vi "initialize.vi"(0 "HGF_Queue":refnum<class "HGF_Queue.lvclass">, 3 "initializationData":variant, 5 "error in (no error)":errorcluster, 7 "binaryString":string, 8 "I8 Array":i8[](array[numeric]), 9 "prependSize? (T)":bool, 11 "byteOrder (0:big-endian, network order)":T1(ring)) -> (14 "dup HGF_Queue":refnum<class "HGF_Queue.lvclass">, 17 "found?":bool, 19 "error out":errorcluster)   [LabVIEW 2014, in "HGF_BaseClasses.lvlib" / "HGF_Queue.lvclass"]
doc: "This is a dynamic dispatch VI to be implemented by child classes to initialize their attributes.\n\n<B>Recommendation:</B> Use Variant for initialization data."
uses:
  HGF_Queue.lvclass
  HGF_TriggeredEvent/HGF_TriggeredEvent.lvclass
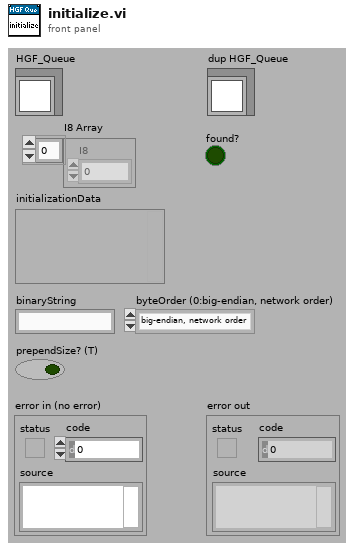
[diagram p1: front panel]
types:
  T1 = enum16{"big-endian, network order", "native, host order", "little-endian"}
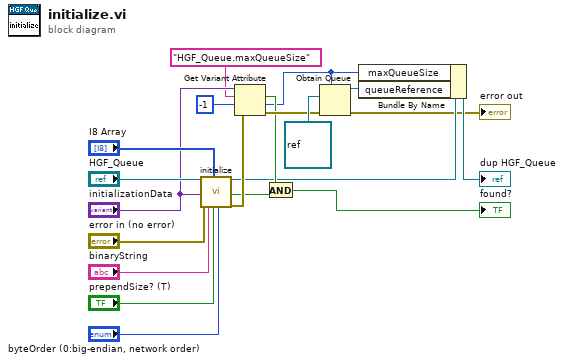
[diagram p0: block diagram]
diagram:
  n1 = call-parent "initialize.vi"("HGF_Timing"="HGF_Queue", "initializationData"="initializationData", "error in (no error)"="error in (no error)", "binaryString"="binaryString", "I8 Array"="I8 Array", "prependSize? (T)"="prependSize? (T)", "byteOrder (0:big-endian, network order)"="byteOrder (0:big-endian, network order)") -> ("dup HGF_Timing"=w8:refnum<class "HGF_Queue.lvclass">, "found?"=w10:bool, "error out"=w16:errorcluster)  [unwired: 1 in, 9 out]
  n2 = Get Variant Attribute(Variant="initializationData", name="HGF_Queue.maxQueueSize", default value (empty Variant)=-1 ("max queue size (-1, unlimited)"), error in=w16) -> (found=w11:bool, value=w5:i32, error out=w15:errorcluster)  [unwired: 1 out]
  n3 = And(x=w11, y=w10) -> (x .and. y?=→"found?":bool)
  n4 = Obtain Queue(max queue size (-1, unlimited)=w5, element data type=refnum<class> refnum ("LabVIEW Object"), error in (no error)=w15) -> (queue out=w6:refnum<queue>, error out=→"error out":errorcluster)  [unwired: 1 in, 2 out]
  n5 = Bundle By Name(cluster=w8, "maxQueueSize"=w5, "queueReference"=w6) -> (→"dup HGF_Queue":refnum<class "HGF_Queue.lvclass">)
